vi "WPI_DMAStreamOffsetsGlobal.vi"(8 "Set":bool, 9 "Enable":T1={"AI0_Low"=FALSE, "AI0_High"=FALSE, "AIAveraged0_Low"=FALSE, "AIAveraged0_High"=FALSE, "AI1_Low"=FALSE, "AI1_High"=FALSE, "AIAveraged1_Low"=TRUE, "AIAveraged1_High"=FALSE, "Accumulator0"=FALSE, "Accumulator1"=FALSE, "DI"=FALSE, "AnalogTriggers"=FALSE, "Counters_Low"=FALSE, "Counters_High"=FALSE, "CounterTimers_Low"=FALSE, "CounterTimers_High"=FALSE, "Encoders_Low"=FALSE, "Encoders_High"=FALSE, "EncoderTimers_Low"=FALSE, "EncoderTimers_High"=FALSE}, 10 "Channels":T3(array[cluster])) -> (2 "StreamOffsets":i32[](array[numeric]))   [LabVIEW 2017]
uses:
  <vilib>/Rock Robotics/WPI/DMA/WPI_DMAChannelTypeEnum.ctl
  <vilib>/Rock Robotics/SystemInterfaces/DMA/FPGA_DMAEnable.ctl
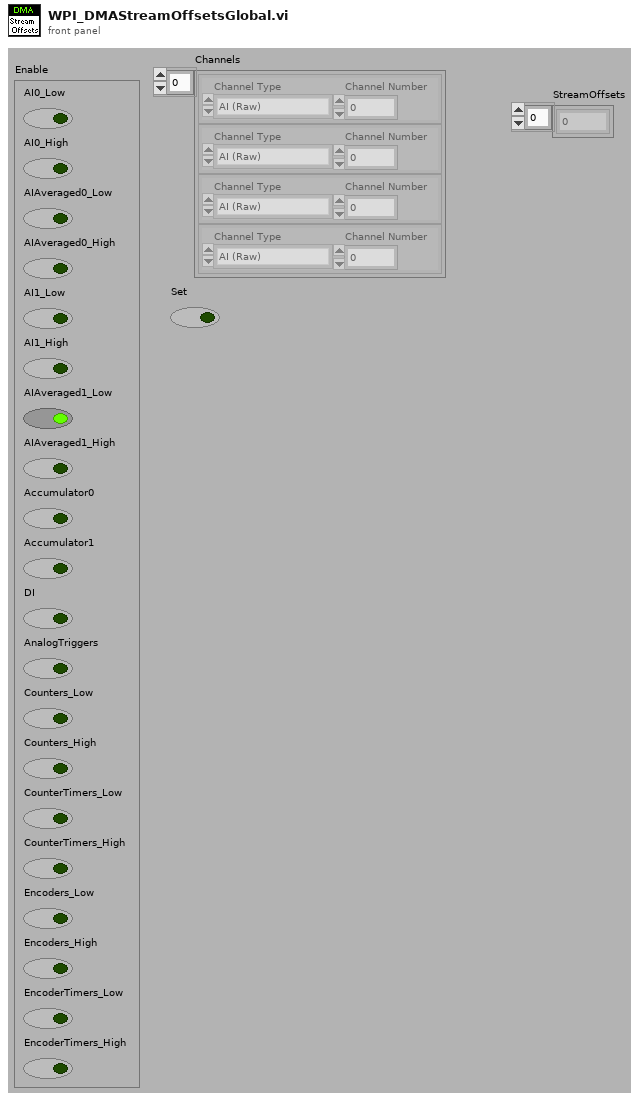
[diagram p1: front panel]
types:
  T1 = typedef "FPGA_DMAEnable.ctl" = cluster{"AI0_Low":bool, "AI0_High":bool, "AIAveraged0_Low":bool, "AIAveraged0_High":bool, "AI1_Low":bool, "AI1_High":bool, "AIAveraged1_Low":bool, "AIAveraged1_High":bool, "Accumulator0":bool, "Accumulator1":bool, "DI":bool, "AnalogTriggers":bool, "Counters_Low":bool, "Counters_High":bool, "CounterTimers_Low":bool, "CounterTimers_High":bool, "Encoders_Low":bool, "Encoders_High":bool, "EncoderTimers_Low":bool, "EncoderTimers_High":bool}
  T2 = typedef "WPI_DMAChannelTypeEnum.ctl" = enum16{"AI (Raw)", "AI (Avg)", "Accumulator", "DI (Raw) Onboard", "DI (Filtered) Onboard", "DI (Raw) MXP", "DI (Filtered) MXP", "Analog Trigger", "Counter", "Counter (Timer)", "Encoder", "Encoder (Timer)", "Time Stamp"}
  T3 = cluster{"Channel Type":T2, "Channel Number":u8}[]
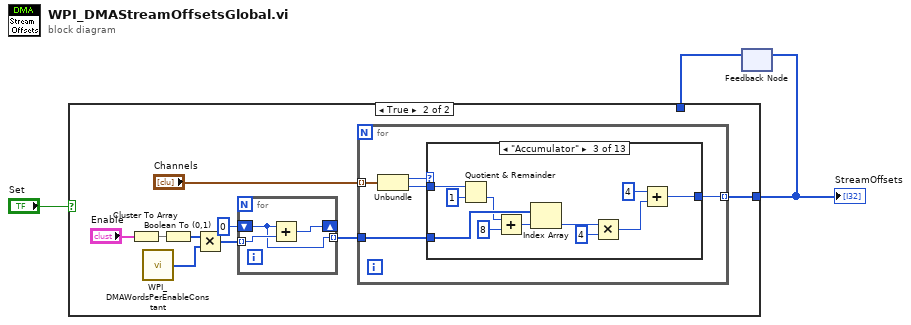
[diagram p0: block diagram]
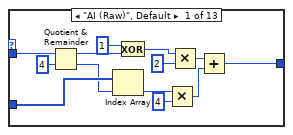
[diagram p3: hidden frame]
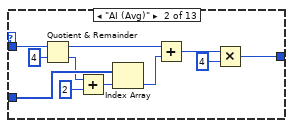
[diagram p4: hidden frame]
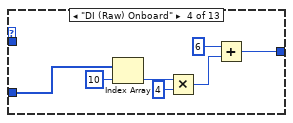
[diagram p5: hidden frame]
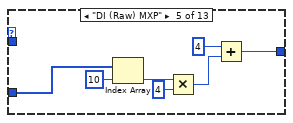
[diagram p6: hidden frame]
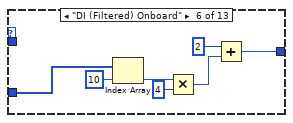
[diagram p7: hidden frame]
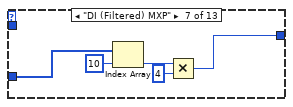
[diagram p8: hidden frame]
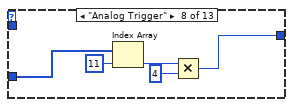
[diagram p9: hidden frame]
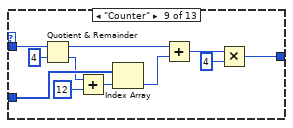
[diagram p10: hidden frame]
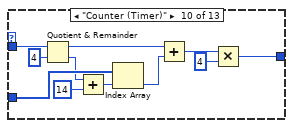
[diagram p11: hidden frame]
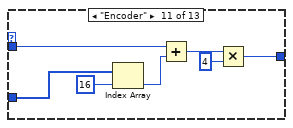
[diagram p12: hidden frame]
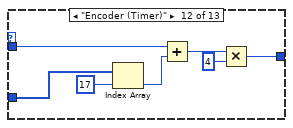
[diagram p13: hidden frame]
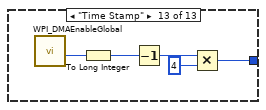
[diagram p14: hidden frame]
diagram:
  n1 = feedback #1() -> (w1:i32[])  [unwired: 1 out]
  n2 = case shown="True" "Set" {
    tunnel: [w4 w6] -> w2
    tunnel: w1 -> [w4 _]
    frame False {
    }
    frame True {
      n3 = Cluster To Array(cluster="Enable") -> (array=w12:bool[])
      n4 = call <vilib>:"WPI_DMAWordsPerEnableConstant.vi"() -> ("WordsPerEnable"=w10:i32[])
      n5 = Boolean To (0,1)(Boolean=w12) -> (0, 1=w11:i16[])
      n6 = Multiply(x=w11, y=w10) -> (x*y=w9:i32[])
      n7 = for {
        tunnel: w9 -> [w128] mode=indexing
        shift-right: [w127] -> _
        shift-left: 0 -> [w126]
        tunnel: [w126] -> w7 mode=indexing
        n8 = Add(x=w126, y=w128) -> (x+y=w127:i32)
      }
      n9 = for {
        tunnel: "Channels" -> [w18] mode=indexing
        tunnel: w7 -> [w15]
        tunnel: [w14] -> w6 mode=indexing
        n10 = Unbundle(w18) -> ("Channel Type"=w17:T2, "Channel Number"=w16:u8)
        n11 = case shown="\"Accumulator\"" w17 {
          tunnel: w16 -> [w30 w41 w52 _ _ _ _ _ w94 w105 w109 w116 _]
          tunnel: w15 -> [w31 w42 w53 w60 w67 w74 w79 w84 w95 w106 w113 w120 _]
          tunnel: [w23 w32 w44 w55 w62 w69 w76 w81 w85 w96 w107 w114 w122] -> w14
          frame "AI (Raw)", Default {
            n12 = Quotient & Remainder(x=w30, y=u8 4) -> (x-y*floor(x/y)=w27:u8, floor(x/y)=w28:u8)
            n13 = Index Array(array=w31, index=w28) -> (element=w24:i32)
            n14 = Exclusive Or(1:w27, 2:u8 1 ("x")) -> (0:w20:u8)
            n15 = Multiply(x=w24, y=4) -> (x*y=w22:i32)
            n16 = Multiply(x=w20, y=2) -> (x*y=w25:i32)
            n17 = Add(x=w25, y=w22) -> (x+y=w23:i32)
          }
          frame "AI (Avg)" {
            n18 = Quotient & Remainder(x=w41, y=u8 4) -> (x-y*floor(x/y)=w34:u8, floor(x/y)=w39:u8)
            n19 = Add(x=w39, y=u8 2) -> (x+y=w37:u8)
            n20 = Index Array(array=w42, index=w37) -> (element=w35:i32)
            n21 = Add(x=w34, y=w35) -> (x+y=w33:i32)
            n22 = Multiply(x=w33, y=4) -> (x*y=w32:i32)
          }
          frame "Accumulator" {
            n23 = Quotient & Remainder(x=w52, y=u8 1) -> (floor(x/y)=w50:u8)  [unwired: 1 out]
            n24 = Add(x=w50, y=u8 8) -> (x+y=w49:u8)
            n25 = Index Array(array=w53, index=w49) -> (element=w47:i32)
            n26 = Multiply(x=w47, y=4 ("x")) -> (x*y=w46:i32)
            n27 = Add(x=4, y=w46) -> (x+y=w44:i32)
          }
          frame "DI (Raw) Onboard" {
            n28 = Index Array(array=w60, index=10) -> (element=w59:i32)
            n29 = Multiply(x=w59, y=4 ("x")) -> (x*y=w57:i32)
            n30 = Add(x=6, y=w57) -> (x+y=w55:i32)
          }
          frame "DI (Raw) MXP" {
            n31 = Index Array(array=w67, index=10) -> (element=w66:i32)
            n32 = Multiply(x=w66, y=4 ("x")) -> (x*y=w64:i32)
            n33 = Add(x=4, y=w64) -> (x+y=w62:i32)
          }
          frame "DI (Filtered) Onboard" {
            n34 = Index Array(array=w74, index=10) -> (element=w73:i32)
            n35 = Multiply(x=w73, y=4 ("x")) -> (x*y=w71:i32)
            n36 = Add(x=2, y=w71) -> (x+y=w69:i32)
          }
          frame "DI (Filtered) MXP" {
            n37 = Index Array(array=w79, index=10) -> (element=w78:i32)
            n38 = Multiply(x=w78, y=4 ("x")) -> (x*y=w76:i32)
          }
          frame "Analog Trigger" {
            n39 = Index Array(array=w84, index=11) -> (element=w83:i32)
            n40 = Multiply(x=w83, y=4) -> (x*y=w81:i32)
          }
          frame "Counter" {
            n41 = Quotient & Remainder(x=w94, y=u8 4) -> (x-y*floor(x/y)=w87:u8, floor(x/y)=w92:u8)
            n42 = Add(x=w92, y=u8 12) -> (x+y=w90:u8)
            n43 = Index Array(array=w95, index=w90) -> (element=w88:i32)
            n44 = Add(x=w87, y=w88) -> (x+y=w86:i32)
            n45 = Multiply(x=w86, y=4) -> (x*y=w85:i32)
          }
          frame "Counter (Timer)" {
            n46 = Quotient & Remainder(x=w105, y=u8 4) -> (x-y*floor(x/y)=w98:u8, floor(x/y)=w103:u8)
            n47 = Add(x=w103, y=u8 14) -> (x+y=w100:u8)
            n48 = Index Array(array=w106, index=w100) -> (element=w101:i32)
            n49 = Add(x=w98, y=w101) -> (x+y=w97:i32)
            n50 = Multiply(x=w97, y=4) -> (x*y=w96:i32)
          }
          frame "Encoder" {
            n51 = Index Array(array=w113, index=u8 16 ("y")) -> (element=w111:i32)
            n52 = Add(x=w109, y=w111) -> (x+y=w108:i32)
            n53 = Multiply(x=w108, y=4) -> (x*y=w107:i32)
          }
          frame "Encoder (Timer)" {
            n54 = Index Array(array=w120, index=u8 17 ("y")) -> (element=w118:i32)
            n55 = Add(x=w116, y=w118) -> (x+y=w115:i32)
            n56 = Multiply(x=w115, y=4) -> (x*y=w114:i32)
          }
          frame "Time Stamp" {
            n57 = call <vilib>:"WPI_DMAEnableGlobal.vi"() -> ("WordsPerSample"=w125:u16)  [unwired: 2 in, 9 out]
            n58 = To Long Integer(number=w125) -> (32bit integer=w123:i32)
            n59 = Decrement(x=w123) -> (x-1=w124:i32)
            n60 = Multiply(x=w124, y=4) -> (x*y=w122:i32)
          }
        }
      }
    }
  }
  "StreamOffsets" <- w2
  n61 = feedback-in #1(w2) -> ()
